vi "PH_Beckhoff_PP_PU.get HV Meas Tagname.vi"(1 "HV Meas Tag":T2, 2 "PU":T1) -> (0 "HV Meas Tagname":string)   [LabVIEW 2014, in "PH_Beckhoff_PP_PU.lvlib"]
doc: "This VI concatenates a Tagname out of strict type def enum controls. It keeps also the information whether the Tag is existing (if not, N/A is given out as name)."
uses:
  PH_Beckhoff_PP_PU.lvlib
  PH_Beckhoff_PP_PU.HV Meas Tags.ctl
  PH_PP_Common/PH_PP_Common.PUs.ctl
  PH_PP_Common/PH_PP_Common.Devices.ctl
  PH_Common/Names/PH_Names.Subsystems.ctl
  PH_Common/Names/PH_Names.Communication Type.ctl
  PH_Common/PH_Common.lvlib
  PH_PP_Common/PH_PP_Common.lvlib
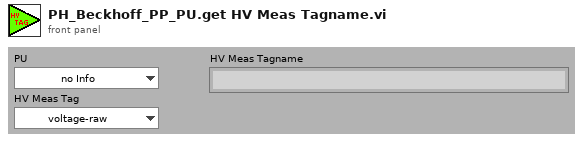
[diagram p1: front panel]
types:
  T1 = typedef "PH_PP_Common.lvlib/PH_PP_Common.PUs.ctl" = enum16{"no Info", "PA-19mm-1", "PA-19mm-2", "PA-45mm-PILC", "PA-45mm-MAIN", "MA-PU-1", "MA-PU-2", "MA-PU-3", "MA-PU-4", "MA-PU-5", "MA-PU-6", "MA-FR", "MA-PILC", "PA-45mm-DP"}
  T2 = typedef "PH_Beckhoff_PP_PU.lvlib/PH_Beckhoff_PP_PU.HV Meas Tags.ctl" = enum16{"voltage-raw", "voltage"}
  T3 = typedef "PH_Common.lvlib/PH_Names.Subsystems.ctl" = enum16{"no Info", "fs-FE", "ns-FE", "PA", "MA", "MAS", "COS", "Exp-LB", "Exp-LL", "PP", "PILS"}
  T4 = typedef "PH_PP_Common.lvlib/PH_PP_Common.Devices.ctl" = enum16{"no Info", "Igni", "RR", "DumpRoss", "PSU", "Trigger", "HV-Meas", "Rods", "Chiller", "Conductivity", "Mercury"}
  T5 = typedef "PH_Common.lvlib/PH_Names.Communication Type.ctl" = enum16{"no Info", "SE", "SA", "AE", "AA", "DE", "DA", "DIM"}
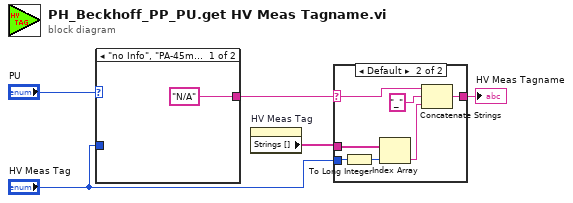
[diagram p0: block diagram]
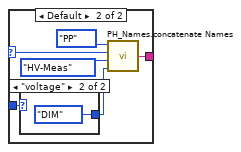
[diagram p2: hidden frame]
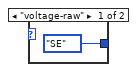
[diagram p3: hidden frame]
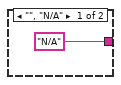
[diagram p4: hidden frame]
diagram:
  n1 = case shown="\"no Info\", \"PA-45mm-PILC\", \"PA-45mm-DP\"" "PU" {
    selector: "PU" -> [_ w11]
    tunnel: ["N/A" ("Subsystem_PU_Devices_Comm Type") w12] -> w4
    tunnel: "HV Meas Tag" -> [_ w7]
    frame "no Info", "PA-45mm-PILC", "PA-45mm-DP" {
    }
    frame Default {
      n2 = case shown="\"voltage\"" w7 {
        tunnel: [PH_Names.Communication_Type."SE" ("Communication Type (no info)") PH_Names.Communication_Type."DIM" ("Communication Type (no info)")] -> w8
        frame "voltage-raw" {
        }
        frame "voltage" {
        }
      }
      n3 = call "PH_Names.concatenate Names.vi"("Communication Type (no info)"=w8, "Devices (no info)"=PH_PP_Common.Devices."HV-Meas", "PU (no info)"=w11, "Subsystem"=PH_Names.Subsystems."PP") -> ("Subsystem_PU_Devices_Comm Type"=w12:string)
    }
  }
  n4 = property on="HV Meas Tag" class="Enum (strict)"() -> ("Strings []"=w3:string[])  [unwired: 2 in, 2 out]
  n5 = case shown="Default" w4 {
    selector: w4 -> [_ w16]
    tunnel: ["N/A" w22] -> w5
    tunnel: w3 -> [_ w21]
    tunnel: "HV Meas Tag" -> [_ w17]
    frame "", "N/A" {
    }
    frame Default {
      n6 = To Long Integer(number=w17) -> (32bit integer=w20:i32)
      n7 = Index Array(array=w21, index=w20) -> (element=w19:string)
      n8 = Concatenate Strings(w16, "_" ("string"), w19) -> (w22:string)
    }
  }
  "HV Meas Tagname" <- w5
